vi "Interpolate.vi"(8 "A (0 -1)":dbl, 10 "High Value":dbl, 11 "Low Value":dbl) -> (2 "Interolated Value":dbl)   [LabVIEW 2018]
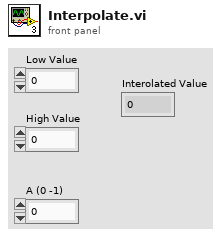
[diagram p1: front panel]
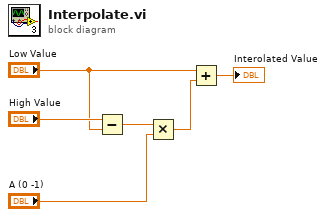
[diagram p0: block diagram]
diagram:
  n1 = Subtract(x="High Value", y="Low Value") -> (x-y=w6:dbl)
  n2 = Multiply(x=w6, y="A (0 -1)") -> (x*y=w4:dbl)
  n3 = Add(x="Low Value", y=w4) -> (x+y=→"Interolated Value":dbl)
